vi "main double species.vi"() -> ()   [LabVIEW 2013]
uses:
  <vilib>/Utility/file.llb/Read From Spreadsheet File (DBL).vi
panel:
  out "Process Index":i8
  out "XY图 4":cluster{i32[], dbl[]}[](graph)
  out "XY图 3":cluster{i32[], dbl[]}[](graph)
  out "OD image 2":dbl[][](graph)
  out "Latest image data 2":dbl[][](array[numeric])
  out "Process Index 2":i8
  out "Two Cameras？":bool
  in  "Fitting Results Save Path 2":string[](array[string])
  in  "Fitting Type 2":u8(ring)
  in  "Force Guess? 2":bool
  in  "Initial guess values 2":dbl[](array[numeric])
  out "From OD fit?":bool
  in  "Current file num":i32
  in  "Fitting Results Save Path":string[](array[string])
  in  "Initial guess values":dbl[](array[numeric])
  out "Latest image data":dbl[][](array[numeric])
  in  "Fitting Type":u8(ring)
  in  "Force Guess?":bool
  out "Fit Done 2":bool
  out "ROI Width 2":u16
  out "ROI Height 2":u16
  out "External Trigger 2":bool
  in  "Fitting Config 2":bool
  in  "Camera Config 2":bool
  in  "Camera2":refnum<k7>(container)
  out "ROI Height":u16
  out "ROI Width":u16
  out "OD image":dbl[][](graph)
  out "External Trigger":bool
  out "XY图":cluster{i32[], dbl[]}[](graph)
  in  "OD fit":bool
  in  "OD num":i32
  out "Fit Done":bool
  in  "Exit":bool
  out "XY图 2":cluster{i32[], dbl[]}[](graph)
  in  "Auto Split":bool
  in  "Fit":bool
  in  "Open File":bool
  in  "Auto Fit":bool
  in  "Stop":bool
  in  "Aquire":bool
  in  "Fitting Config 1":bool
  in  "Camera Config 1":bool
  in  "Initialize":bool
  in  "Camera1":refnum<k7>(container)
  # "Camera Config"
  # "Fitting Config"
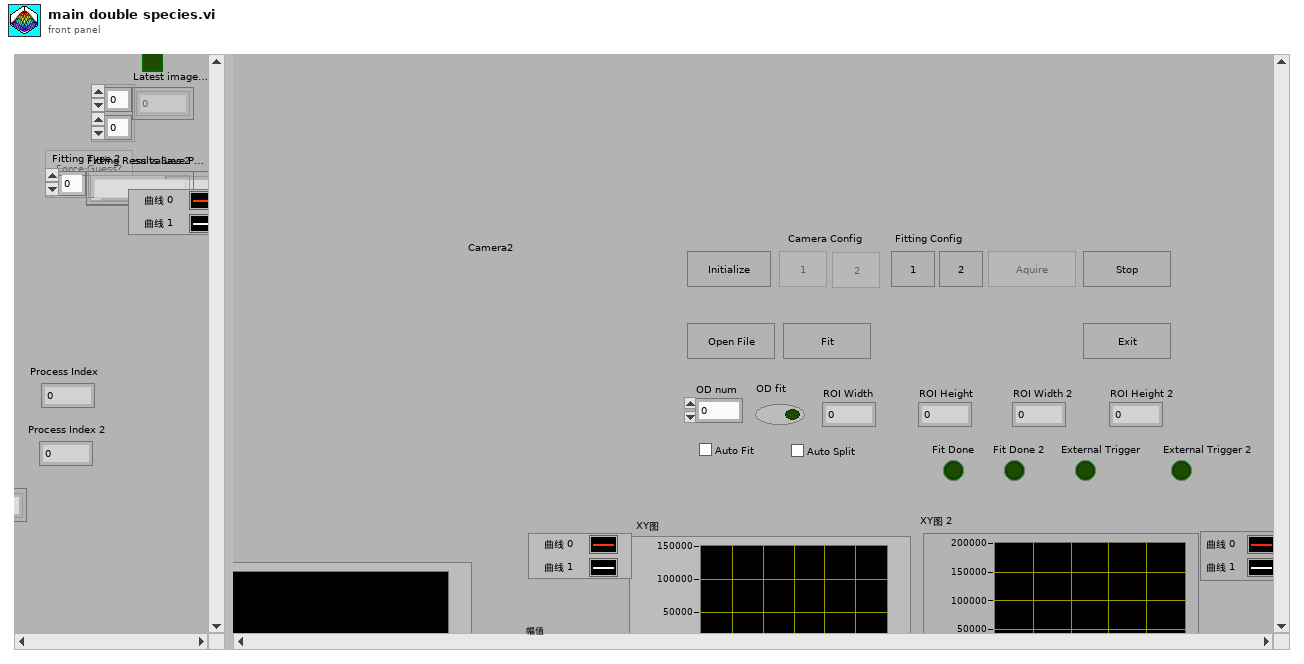
[diagram p1: front panel]
types:
  T1 = enum8{"Enabled", "Disabled", "Disabled and Grayed Out"}
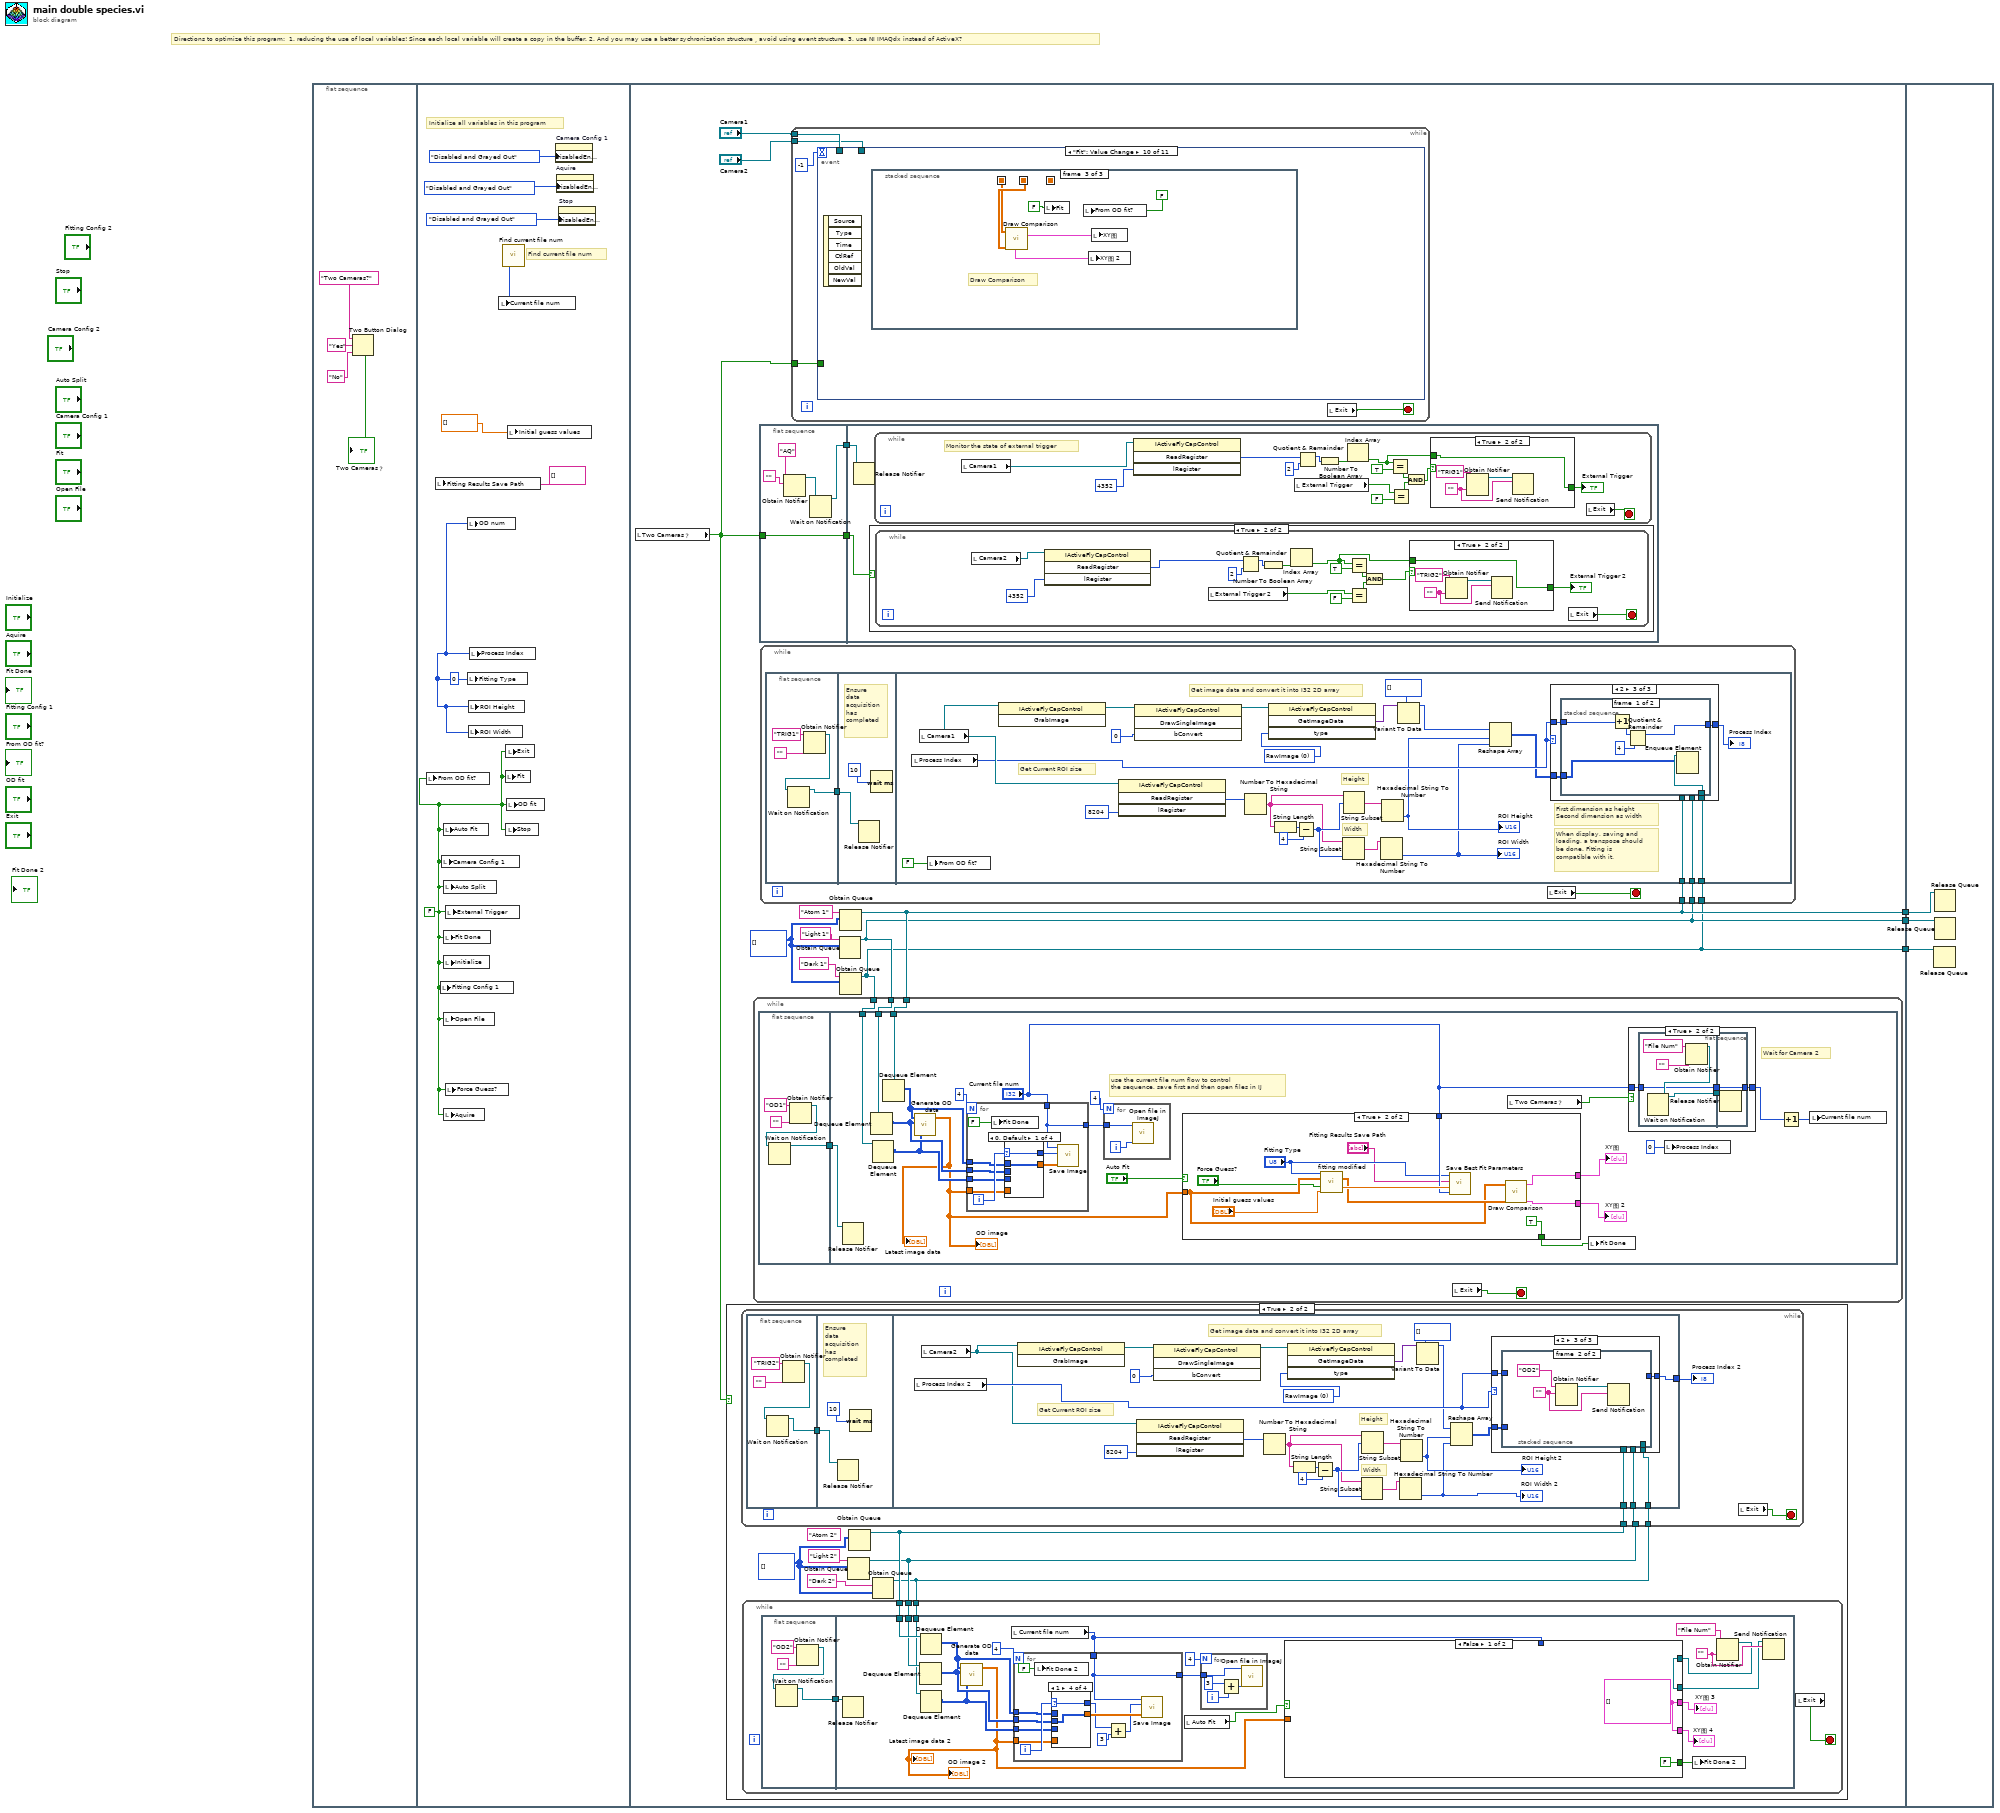
[diagram p0: block diagram]
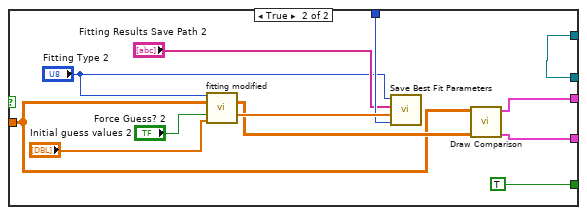
[diagram p3: hidden frame]
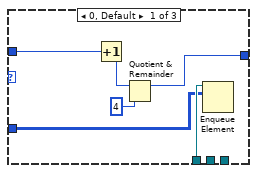
[diagram p7: hidden frame]
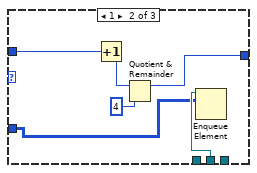
[diagram p8: hidden frame]
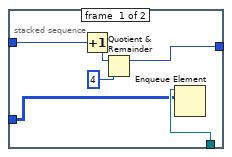
[diagram p9: hidden frame]
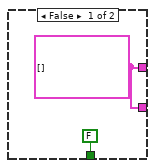
[diagram p11: hidden frame]
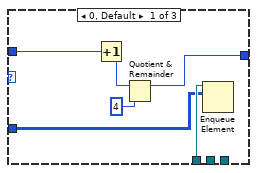
[diagram p18: hidden frame]
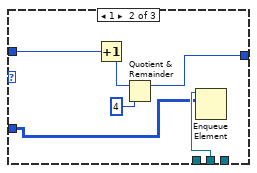
[diagram p19: hidden frame]
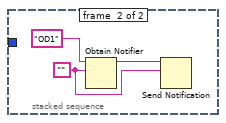
[diagram p20: hidden frame]
diagram:
  # "Directions to optimize this program:  1. reducing the use of local variables! Since each local variable will create a copy in the buffer. 2. And you may use a better sychronization structure，avoid using event structure. 3. use NI IMAQdx instead of ActiveX?"
  n1 = flat-sequence {
    tunnel: [w22] -> w3
    tunnel: [w21] -> w2
    tunnel: [w20] -> w1
    tunnel: w3 -> [w446]
    tunnel: w2 -> [w445]
    tunnel: w1 -> [w444]
    frame #0 {
      n2 = Two Button Dialog(message="Two Cameras?" ("消息"), 1:"No" ("F按钮名称（“取消”）"), 2:"Yes" ("T按钮名称（“确定”）")) -> (T button?=→"Two Cameras？":bool)
    }
    frame #1 {
      w11 = 0 ("OD num")
      w9 = FALSE ("Aquire")
      # "Find current file num"
      # "Initialize all variables in this program"
      n3 = local write "From OD fit?"(w9) -> ()
      n4 = local write "Fitting Results Save Path"(string[] [] ("Fitting Results Save Path")) -> ()
      n5 = local write "Fitting Config 1"(w9) -> ()
      n6 = local write "Camera Config 1"(w9) -> ()
      n7 = local write "Auto Fit"(w9) -> ()
      n8 = local write "Auto Split"(w9) -> ()
      n9 = local write "Fit Done"(w9) -> ()
      n10 = local write "Initialize"(w9) -> ()
      n11 = local write "Open File"(w9) -> ()
      n12 = local write "Aquire"(w9) -> ()
      n13 = local write "Force Guess?"(w9) -> ()
      n14 = local write "External Trigger"(w9) -> ()
      n15 = local write "OD num"(w11) -> ()
      n16 = local write "Fitting Type"(w11) -> ()
      n17 = local write "ROI Height"(w11) -> ()
      n18 = local write "ROI Width"(w11) -> ()
      n19 = local write "Process Index"(w11) -> ()
      n20 = call "Find current file num.vi"() -> ("Current File Num"=w8:u16)  [unwired: 2 in]
      n21 = local write "Current file num"(w8) -> ()
      n22 = local write "Fit"(w9) -> ()
      n23 = local write "Exit"(w9) -> ()
      n24 = local write "Stop"(w9) -> ()
      n25 = local write "OD fit"(w9) -> ()
      n26 = local write "Initial guess values"(dbl[] [] ("Best fit parameters")) -> ()
      n27 = property on="Camera Config 1" class="Bool (strict)"("DisabledEnum"=T1."Disabled and Grayed Out" ("禁用")) -> ()  [unwired: 2 in, 2 out]
      n28 = property on="Aquire" class="Bool (strict)"("DisabledEnum"=T1."Disabled and Grayed Out" ("禁用")) -> ()  [unwired: 2 in, 2 out]
      n29 = property on="Stop" class="Bool (strict)"("DisabledEnum"=T1."Disabled and Grayed Out" ("禁用")) -> ()  [unwired: 2 in, 2 out]
    }
    frame #2 {
      w23 = u16[][] [] ("输出数组")
      n30 = local read "Two Cameras？"() -> (w16:bool)
      n31 = case shown="True" w16 {
        frame False {
        }
        frame True {
          w31 = u16[][] [] ("输出数组")
          (unwired) "Atom 2" ("名称（未命名）")
          n32 = Obtain Queue(name (unnamed)="Light 2" ("名称（未命名）"), element data type=w31) -> (queue out=w29:refnum<queue>)  [unwired: 3 in, 2 out]
          n33 = Obtain Queue(element data type=w31) -> (queue out=w30:refnum<queue>)  [unwired: 4 in, 2 out]
          n34 = Obtain Queue(name (unnamed)="Dark 2" ("名称（未命名）"), element data type=w31) -> (queue out=w28:refnum<queue>)  [unwired: 3 in, 2 out]
          n35 = while {
            tunnel: w30 -> [w103]
            tunnel: w29 -> [w102]
            tunnel: w28 -> [w101]
            stop <- w104 stop-if-true
            n36 = flat-sequence {
              tunnel: [w107] -> w106
              tunnel: w106 -> [w111]
              tunnel: [w122] -> w105
              tunnel: w103 -> [w115]
              tunnel: w102 -> [w114]
              tunnel: w101 -> [w113]
              frame #0 {
                n37 = Obtain Notifier(name (unnamed)="TRIG2" ("名称（未命名）"), notification data type="") -> (notifier out=w108:refnum<notifier>)  [unwired: 2 in, 2 out]
                n38 = Wait on Notification(notifier=w108) -> (notifier out=w107:refnum<notifier>)  [unwired: 3 in, 3 out]
              }
              frame #1 {
                # "Ensure\ndata\nacquisition\nhas \ncompleted"
                n39 = Release Notifier(notifier=w111) -> ()  [unwired: 2 in, 3 out]
                n40 = Wait (ms)(milliseconds to wait=u32 10 ("等待时间（毫秒）")) -> ()  [unwired: 1 out]
              }
              frame #2 {
                w136 = 0 items=["RawImage", "ColorProcessedImage"] ("type")
                # "Get image data and convert it into I32 2D array"
                # "Width"
                # "Height"
                # "Get Current ROI size"
                n41 = local read "Process Index 2"() -> (w121:i8)
                n42 = local read "Camera2"() -> (w116:refnum<k7>)
                n43 = invoke class="IActiveFlyCapControl" method="GrabImage"(reference=w116) -> (reference out=w125:refnum<k7>)  [unwired: 2 in, 2 out]
                n44 = invoke class="IActiveFlyCapControl" method="ReadRegister"(reference=w116, "lRegister"=u32 8204) -> ("ReadRegister"=w133:u32)  [unwired: 2 in, 3 out]
                n45 = invoke class="IActiveFlyCapControl" method="DrawSingleImage"(reference=w125, "bConvert"=0) -> (reference out=w126:refnum<k7>)  [unwired: 2 in, 3 out]
                n46 = Number To Hexadecimal String(2:w133) -> (0:w129:string)  [unwired: 1 in]
                n47 = invoke class="IActiveFlyCapControl" method="GetImageData"(reference=w126, "type"=w136) -> ("GetImageData"=w134:variant)  [unwired: 2 in, 3 out]
                n48 = String Length(string=w129) -> (length=w132:i32)
                n49 = Subtract(x=w132, y=4) -> (x-y=w130:i32)
                n50 = String Subset(string=w129, length (rest)=w130) -> (substring=w127:string)  [unwired: 1 in]
                n51 = String Subset(string=w129, offset (0)=w130) -> (substring=w128:string)  [unwired: 1 in]
                n52 = Hexadecimal String To Number(string=w127) -> (number=w119:u32)  [unwired: 2 in, 1 out]
                "ROI Width 2" <- w119
                n53 = Hexadecimal String To Number(string=w128) -> (number=w120:u32)  [unwired: 2 in, 1 out]
                "ROI Height 2" <- w120
                n54 = Variant To Data(type=u16[] [], Variant=w134) -> (data=w118:u16[])  [unwired: 1 in, 1 out]
                n55 = Reshape Array(w118, w120, w119) -> (w117:u16[][])
                n56 = case shown="2" w121 {
                  tunnel: w121 -> [w140 w146 w152]
                  tunnel: w117 -> [w138 w144 w151]
                  tunnel: w115 -> [w139 _ _]
                  tunnel: w114 -> [_ w145 _]
                  tunnel: w113 -> [_ _ w150]
                  tunnel: [w137 w143 w149] -> w122
                  frame 0, Default {
                    n57 = Increment(x=w140) -> (x+1=w141:i8)
                    n58 = Quotient & Remainder(x=w141, y=4) -> (x-y*floor(x/y)=w137:i32)  [unwired: 1 out]
                    n59 = Enqueue Element(queue=w139, element=w138) -> ()  [unwired: 2 in, 3 out]
                  }
                  frame 1 {
                    n60 = Increment(x=w146) -> (x+1=w147:i8)
                    n61 = Quotient & Remainder(x=w147, y=4) -> (x-y*floor(x/y)=w143:i32)  [unwired: 1 out]
                    n62 = Enqueue Element(queue=w145, element=w144) -> ()  [unwired: 2 in, 3 out]
                  }
                  frame 2 {
                    n63 = stacked-sequence {
                      tunnel: w152 -> [w156 _]
                      tunnel: w151 -> [w154 _]
                      tunnel: w150 -> [w155 _]
                      tunnel: [w153 _] -> w149
                      frame #0 {
                        n64 = Increment(x=w156) -> (x+1=w157:i8)
                        n65 = Quotient & Remainder(x=w157, y=4) -> (x-y*floor(x/y)=w153:i32)  [unwired: 1 out]
                        n66 = Enqueue Element(queue=w155, element=w154) -> ()  [unwired: 2 in, 3 out]
                      }
                      frame #1 {
                        w159 = ""
                        n67 = Obtain Notifier(name (unnamed)="OD2" ("名称（未命名）"), notification data type=w159) -> (notifier out=w161:refnum<notifier>)  [unwired: 2 in, 2 out]
                        n68 = Send Notification(notification=w159, notifier=w161) -> ()  [unwired: 1 in, 2 out]
                      }
                    }
                  }
                }
              }
            }
            n69 = local read "Exit"() -> (w104:bool)
            "Process Index 2" <- w105
          }
          n70 = while {
            tunnel: w30 -> [w37]
            tunnel: w29 -> [w36]
            tunnel: w28 -> [w35]
            stop <- w34 stop-if-true
            n71 = flat-sequence {
              tunnel: [w39] -> w38
              tunnel: w38 -> [w62]
              tunnel: w37 -> [w57]
              tunnel: w36 -> [w56]
              tunnel: w35 -> [w55]
              frame #0 {
                n72 = Obtain Notifier(name (unnamed)="OD2" ("名称（未命名）"), notification data type="") -> (notifier out=w40:refnum<notifier>)  [unwired: 2 in, 2 out]
                n73 = Wait on Notification(notifier=w40) -> (notifier out=w39:refnum<notifier>)  [unwired: 3 in, 3 out]
              }
              frame #1 {
                w46 = ""
                n74 = Release Notifier(notifier=w62) -> ()  [unwired: 2 in, 3 out]
                n75 = Dequeue Element(queue=w56) -> (element=w59:u16[][])  [unwired: 2 in, 3 out]
                n76 = Dequeue Element(queue=w57) -> (element=w60:u16[][])  [unwired: 2 in, 3 out]
                n77 = Dequeue Element(queue=w55) -> (element=w58:u16[][])  [unwired: 2 in, 3 out]
                n78 = call "Generate OD data.vi"("dark"=w58, "light"=w59, "atom"=w60) -> ("OD image"=w52:dbl[][])  [unwired: 3 in]
                "Latest image data 2" <- w52
                "OD image 2" <- w52
                n79 = local read "Current file num"() -> (w50:i32)
                n80 = for {
                  N: 4 -> [_]
                  tunnel: w60 -> [w91]
                  tunnel: w59 -> [w90]
                  tunnel: w58 -> [w89]
                  tunnel: w52 -> [w88]
                  tunnel: w50 -> [w86]
                  tunnel: [w86] -> w53
                  i -> [w92]
                  n81 = local write "Fit Done 2"(FALSE ("Fit Done 2")) -> ()
                  n82 = case shown="1" w92 {
                    selector: w92 -> [w94 w96 w98 w100]
                    tunnel: w91 -> [w93 _ _ _]
                    tunnel: w90 -> [_ _ _ w99]
                    tunnel: w89 -> [_ w95 _ _]
                    tunnel: w88 -> [_ _ w97 _]
                    tunnel: [w94 w96 w98 w100] -> w85
                    tunnel: [w93 w95 w97 w99] -> w87
                    frame 0, Default {
                    }
                    frame 2 {
                    }
                    frame 3 {
                    }
                    frame 1 {
                    }
                  }
                  n83 = Add(x=w85, y=3 ("x")) -> (x+y=w84:i32)
                  n84 = call "Save Image.vi"("Data"=w87, "Process Index"=w84, "Current File Num"=w86) -> ()  [unwired: 9 in]
                }
                n85 = local read "Auto Fit"() -> (w51:bool)
                n86 = for {
                  N: 4 -> [_]
                  tunnel: w53 -> [w81]
                  i -> [w79]
                  n87 = Add(x=i8 3, y=w79) -> (x+y=w78:i32)
                  n88 = call "Open file in ImageJ.vi"("Process Index"=w78, "Current File Num"=w81) -> ()  [unwired: 10 in]
                }
                n89 = Obtain Notifier(name (unnamed)="File Num" ("名称（未命名）"), notification data type=w46) -> (notifier out=w45:refnum<notifier>)  [unwired: 2 in, 2 out]
                n90 = case shown="False" w51 {
                  tunnel: w52 -> [_ w74]
                  tunnel: w50 -> [_ w76]
                  tunnel: [w65 w73] -> w49
                  tunnel: [w65 w72] -> w48
                  tunnel: w45 -> [w64 w67]
                  tunnel: [w64 w67] -> w44
                  tunnel: [FALSE ("Fit Done 2") TRUE ("Fit Done 2")] -> w43
                  frame False {
                    w65 = cluster{i32[], dbl[]}[] [] ("Horizontal Comparison")
                  }
                  frame True {
                    n91 = call "fitting modified.vi"("fitting type"="Fitting Type 2", "2D data"=w74, "force guess?"="Force Guess? 2", "intial guess value"="Initial guess values 2") -> ("best fit"=w75:dbl[][], "best fit parameters"=w77:dbl[])  [unwired: 9 in, 1 out]
                    n92 = call "Save Best Fit Parameters.vi"("Current File Num"=w76, "Best Fit Parameters"=w77, "Fitting Results Save Path"="Fitting Results Save Path 2", "Fitting Type"="Fitting Type 2") -> ()  [unwired: 8 in]
                    n93 = call "Draw Comparison.vi"("Best Fit"=w75, "Raw Data"=w74) -> ("Vertical Comparison"=w72:cluster{i32[], dbl[]}[], "Horizontal Comparison"=w73:cluster{i32[], dbl[]}[])  [unwired: 7 in]
                  }
                }
                "XY图 3" <- w49
                "XY图 4" <- w48
                n94 = local write "Fit Done 2"(w43) -> ()
                n95 = Send Notification(notification=w46, notifier=w44) -> ()  [unwired: 1 in, 2 out]
              }
            }
            n96 = local read "Exit"() -> (w34:bool)
          }
        }
      }
      n97 = flat-sequence {
        tunnel: [w236] -> w27
        tunnel: w16 -> [w235]
        tunnel: [w235] -> w17
        tunnel: w27 -> [w241]
        tunnel: w17 -> [w240]
        frame #0 {
          n98 = Obtain Notifier(name (unnamed)="AQ" ("名称（未命名）"), notification data type="") -> (notifier out=w238:refnum<notifier>)  [unwired: 2 in, 2 out]
          n99 = Wait on Notification(notifier=w238) -> (notifier out=w236:refnum<notifier>)  [unwired: 3 in, 3 out]
        }
        frame #1 {
          n100 = Release Notifier(notifier=w241) -> ()  [unwired: 2 in, 3 out]
          n101 = case shown="True" w240 {
            frame False {
            }
            frame True {
              n102 = while {
                stop <- w256 stop-if-true
                n103 = local read "Camera2"() -> (w242:refnum<k7>)
                n104 = invoke class="IActiveFlyCapControl" method="ReadRegister"(reference=w242, "lRegister"=u32 4352) -> ("ReadRegister"=w243:u32)  [unwired: 2 in, 3 out]
                n105 = local read "External Trigger 2"() -> (w245:bool)
                n106 = Quotient & Remainder(x=w243, y=u32 2) -> (x-y*floor(x/y)=w249:u32)  [unwired: 1 out]
                n107 = Number To Boolean Array(number=w249) -> (Boolean array=w248:bool[])
                n108 = Index Array(array=w248) -> (element=w247:bool)  [unwired: 1 in]
                n109 = Equal?(x=w247, y=TRUE) -> (x = y?=w252:bool)
                n110 = Equal?(x=w245, y=FALSE) -> (x = y?=w253:bool)
                n111 = And(x=w252, y=w253) -> (x .and. y?=w251:bool)
                n112 = case shown="True" w251 {
                  tunnel: w247 -> [w257 w258]
                  tunnel: [w257 w258] -> w246
                  frame False {
                  }
                  frame True {
                    w259 = ""
                    n113 = Obtain Notifier(name (unnamed)="TRIG2" ("名称（未命名）"), notification data type=w259) -> (notifier out=w260:refnum<notifier>)  [unwired: 2 in, 2 out]
                    n114 = Send Notification(notification=w259, notifier=w260) -> ()  [unwired: 1 in, 2 out]
                  }
                }
                "External Trigger 2" <- w246
                n115 = local read "Exit"() -> (w256:bool)
              }
            }
          }
          n116 = while {
            stop <- w276 stop-if-true
            # "Monitor the state of external trigger"
            n117 = local read "Camera1"() -> (w275:refnum<k7>)
            n118 = invoke class="IActiveFlyCapControl" method="ReadRegister"(reference=w275, "lRegister"=u32 4352) -> ("ReadRegister"=w273:u32)  [unwired: 2 in, 3 out]
            n119 = local read "External Trigger"() -> (w268:bool)
            n120 = Quotient & Remainder(x=w273, y=u32 2) -> (x-y*floor(x/y)=w271:u32)  [unwired: 1 out]
            n121 = Number To Boolean Array(number=w271) -> (Boolean array=w270:bool[])
            n122 = Index Array(array=w270) -> (element=w263:bool)  [unwired: 1 in]
            n123 = Equal?(x=w263, y=TRUE) -> (x = y?=w265:bool)
            n124 = Equal?(x=w268, y=FALSE) -> (x = y?=w266:bool)
            n125 = And(x=w265, y=w266) -> (x .and. y?=w264:bool)
            n126 = case shown="True" w264 {
              tunnel: w263 -> [w277 w278]
              tunnel: [w277 w278] -> w262
              frame False {
              }
              frame True {
                w279 = ""
                n127 = Obtain Notifier(name (unnamed)="TRIG1" ("名称（未命名）"), notification data type=w279) -> (notifier out=w280:refnum<notifier>)  [unwired: 2 in, 2 out]
                n128 = Send Notification(notification=w279, notifier=w280) -> ()  [unwired: 1 in, 2 out]
              }
            }
            "External Trigger" <- w262
            n129 = local read "Exit"() -> (w276:bool)
          }
        }
      }
      n130 = while {
        tunnel: "Camera1" -> [w346]
        tunnel: "Camera2" -> [w345]
        tunnel: w16 -> [w343]
        stop <- w347 stop-if-true
        n131 = event shown="[9] \"Fit\": Value Change" {
          selector: _ -> [_ _ _ _ _ _ _ _ _ _ _]
          dyn-events: _ -> [_ _ _ _ _ _ _ _ _ _ _]
          timeout: -1 -> [_ _ _ _ _ _ _ _ _ _ _]
          tunnel: w346 -> [_ w355 w374 _ _ _ _ w396 w411 _ _]
          tunnel: w345 -> [_ w354 _ w377 _ _ _ w397 w413 _ _]
          tunnel: w343 -> [_ w352 _ w376 _ w386 _ w394 w409 _ _]
          event "OD fit": Value Change {
            n132 = event-data() -> ()  [unwired: 1 in, 6 out]
            n133 = local write "OD fit"(FALSE ("OD fit")) -> ()
            n134 = call "Read OD data.vi"("OD num"="OD num") -> ("OD data"=w349:dbl[][])  [unwired: 4 in]
            n135 = local write "Latest image data"(w349) -> ()
            n136 = local write "OD image"(w349) -> ()
            n137 = local write "From OD fit?"(TRUE ("From OD fit?")) -> ()
          }
          event "Initialize": Value Change {
            w361 = 2 items=["FreeRunning", "LockNext", "LockLatest"] ("mode")
            # "Setup Camera Index"
            # "Set grab mode"
            # "Make Sure the camera is not running"
            n138 = event-data() -> ()  [unwired: 1 in, 6 out]
            n139 = case shown="True" w352 {
              tunnel: w354 -> [_ w369]
              frame False {
              }
              frame True {
                w366 = 2 items=["FreeRunning", "LockNext", "LockLatest"] ("mode")
                n140 = property class="IActiveFlyCapControl"(reference=w369, "Camera"=u32 1) -> (reference out=w368:refnum<k7>)  [unwired: 1 in, 1 out]
                n141 = invoke class="IActiveFlyCapControl" method="ShowCamSlnModal"(reference=w368) -> (reference out=w367:refnum<k7>)  [unwired: 2 in, 2 out]
                n142 = property class="IActiveFlyCapControl"(reference=w367, "Start"=0 ("Camera")) -> (reference out=w371:refnum<k7>)  [unwired: 1 in, 1 out]
                n143 = invoke class="IActiveFlyCapControl" method="SetGrabMode"(reference=w371, "mode"=w366) -> (reference out=w365:refnum<k7>)  [unwired: 2 in, 3 out]
                n144 = local write "Camera2"(w365) -> ()
              }
            }
            n145 = property class="IActiveFlyCapControl"(reference=w355, "Camera"=u32 0) -> (reference out=w360:refnum<k7>)  [unwired: 1 in, 1 out]
            n146 = invoke class="IActiveFlyCapControl" method="ShowCamSlnModal"(reference=w360) -> (reference out=w358:refnum<k7>)  [unwired: 2 in, 2 out]
            n147 = property class="IActiveFlyCapControl"(reference=w358, "Start"=0 ("Camera")) -> (reference out=w357:refnum<k7>)  [unwired: 1 in, 1 out]
            n148 = invoke class="IActiveFlyCapControl" method="SetGrabMode"(reference=w357, "mode"=w361) -> (reference out=w353:refnum<k7>)  [unwired: 2 in, 3 out]
            n149 = local write "Camera1"(w353) -> ()
            n150 = property on="Camera Config 1" class="Bool (strict)"("DisabledEnum"=T1."Enabled" ("禁用")) -> ()  [unwired: 2 in, 2 out]
            n151 = local write "Initialize"(FALSE ("Initialize")) -> ()
            n152 = property on="Aquire" class="Bool (strict)"("DisabledEnum"=T1."Enabled" ("禁用")) -> ()  [unwired: 2 in, 2 out]
          }
          event "Camera Config 1": Value Change {
            n153 = event-data() -> ()  [unwired: 1 in, 6 out]
            n154 = invoke class="IActiveFlyCapControl" method="ToggleCamCtlDlg"(reference=w374) -> (reference out=w373:refnum<k7>)  [unwired: 2 in, 2 out]
            n155 = local write "Camera Config 1"(FALSE ("Camera Config")) -> ()
            n156 = local write "Camera1"(w373) -> ()
          }
          event "Camera Config 2": Value Change {
            n157 = event-data() -> ()  [unwired: 1 in, 6 out]
            n158 = case shown="True" w376 {
              tunnel: w377 -> [_ w379]
              frame False {
              }
              frame True {
                n159 = invoke class="IActiveFlyCapControl" method="ToggleCamCtlDlg"(reference=w379) -> (reference out=w378:refnum<k7>)  [unwired: 2 in, 2 out]
                n160 = local write "Camera Config 2"(FALSE ("Camera Config 2")) -> ()
                n161 = local write "Camera2"(w378) -> ()
              }
            }
          }
          event "Fitting Config 1": Value Change {
            # "pump out fitting config. and transfer parameters"
            n162 = event-data() -> ()  [unwired: 1 in, 6 out]
            n163 = call "Fitting Configuration.vi"() -> ("intial guess"=w381:dbl[], "Force Guess？"=w382:bool, "Fitting Type"=w384:u16, "Fitting Results Save Path"=w383:string[])  [unwired: 5 in]
            n164 = local write "Fitting Results Save Path"(w383) -> ()
            n165 = local write "Fitting Type"(w384) -> ()
            n166 = local write "Fitting Config 1"(FALSE ("Fitting Config")) -> ()
            n167 = local write "Initial guess values"(w381) -> ()
            n168 = local write "Force Guess?"(w382) -> ()
          }
          event "Fitting Config 2": Value Change {
            n169 = event-data() -> ()  [unwired: 1 in, 6 out]
            n170 = case shown="True" w386 {
              frame False {
              }
              frame True {
                n171 = call "Fitting Configuration 2.vi"() -> ("intial guess"=w388:dbl[], "Force Guess？"=w389:bool, "Fitting Type"=w390:u16, "Fitting Results Save Path"=w391:string[])  [unwired: 5 in]
                n172 = local write "Initial guess values 2"(w388) -> ()
                n173 = local write "Force Guess? 2"(w389) -> ()
                n174 = local write "Fitting Results Save Path 2"(w391) -> ()
                n175 = local write "Fitting Type 2"(w390) -> ()
              }
            }
            n176 = local write "Fitting Config 2"(FALSE ("Fitting Config 2")) -> ()
          }
          event "Open File": Value Change {
            n177 = event-data() -> ()  [unwired: 1 in, 6 out]
            n178 = call-poly <vilib>:"Read From Spreadsheet File.vi"() -> ("all rows"=w392:dbl[][])  [unwired: 7 in, 4 out]
            n179 = local write "Open File"(FALSE ("Open File")) -> ()
            n180 = local write "OD image"(w392) -> ()
            n181 = local write "Latest image data"(w392) -> ()
          }
          event "Aquire": Value Change {
            w398 = 1 ("Start")
            w399 = ""
            # "Start the camera"
            n182 = event-data() -> ()  [unwired: 1 in, 6 out]
            n183 = case shown="True" w394 {
              tunnel: w398 -> [_ w408]
              tunnel: w397 -> [_ w407]
              frame False {
              }
              frame True {
                n184 = property class="IActiveFlyCapControl"(reference=w407, "Start"=w408) -> (reference out=w406:refnum<k7>)  [unwired: 1 in, 1 out]
                n185 = local write "Camera2"(w406) -> ()
              }
            }
            n186 = property class="IActiveFlyCapControl"(reference=w396, "Start"=w398) -> (reference out=w395:refnum<k7>)  [unwired: 1 in, 1 out]
            n187 = Obtain Notifier(name (unnamed)="AQ" ("名称（未命名）"), notification data type=w399) -> (notifier out=w400:refnum<notifier>)  [unwired: 2 in, 2 out]
            n188 = Send Notification(notification=w399, notifier=w400) -> ()  [unwired: 1 in, 2 out]
            n189 = local write "Camera1"(w395) -> ()
            n190 = property on="Aquire" class="Bool (strict)"("DisabledEnum"=T1."Disabled and Grayed Out" ("禁用")) -> ()  [unwired: 2 in, 2 out]
            n191 = property on="Stop" class="Bool (strict)"("DisabledEnum"=T1."Enabled" ("禁用")) -> ()  [unwired: 2 in, 2 out]
            n192 = property on="Camera Config 1" class="Bool (strict)"("DisabledEnum"=T1."Disabled and Grayed Out" ("禁用")) -> ()  [unwired: 2 in, 2 out]
            n193 = local write "Aquire"(FALSE ("Initialize")) -> ()
          }
          event "Stop": Value Change {
            w412 = 0 ("Start")
            # "stop the camera"
            n194 = event-data() -> ()  [unwired: 1 in, 6 out]
            n195 = case shown="True" w409 {
              tunnel: w413 -> [_ w419]
              tunnel: w412 -> [_ w418]
              frame False {
              }
              frame True {
                n196 = property class="IActiveFlyCapControl"(reference=w419, "Start"=w418) -> (reference out=w417:refnum<k7>)  [unwired: 1 in, 1 out]
                n197 = local write "Camera2"(w417) -> ()
              }
            }
            n198 = property class="IActiveFlyCapControl"(reference=w411, "Start"=w412) -> (reference out=w410:refnum<k7>)  [unwired: 1 in, 1 out]
            n199 = local write "Camera1"(w410) -> ()
            n200 = local write "Stop"(FALSE ("Initialize")) -> ()
            n201 = property on="Stop" class="Bool (strict)"("DisabledEnum"=T1."Disabled and Grayed Out" ("禁用")) -> ()  [unwired: 2 in, 2 out]
            n202 = property on="Aquire" class="Bool (strict)"("DisabledEnum"=T1."Enabled" ("禁用")) -> ()  [unwired: 2 in, 2 out]
          }
          event "Fit": Value Change {
            n203 = event-data() -> ()  [unwired: 1 in, 6 out]
            n204 = stacked-sequence {
              seq-local: [w421 _ _] -> [_ _ w440]
              seq-local: [w422 _ _] -> [_ _ w438]
              seq-local: [w420 _ _] -> [_ w431 _]
              frame #0 {
                n205 = flat-sequence {
                  tunnel: [w425] -> w422
                  tunnel: [w424] -> w421
                  tunnel: [w423] -> w420
                  frame #0 {
                    # "Fit the latest data"
                    n206 = local read "Latest image data"() -> (w425:dbl[][])
                    n207 = local read "Initial guess values"() -> (w427:dbl[])
                    n208 = local read "Force Guess?"() -> (w428:bool)
                    n209 = local read "Fitting Type"() -> (w426:u8)
                    n210 = call "fitting modified.vi"("fitting type"=w426, "2D data"=w425, "force guess?"=w428, "intial guess value"=w427) -> ("best fit"=w424:dbl[][], "best fit parameters"=w423:dbl[])  [unwired: 9 in, 1 out]
                  }
                  frame #1 {
                    n211 = local write "Fit"(FALSE ("Fit")) -> ()
                    n212 = local write "Fit Done"(TRUE ("Fit Done")) -> ()
                  }
                }
              }
              frame #1 {
                # "Save best fit parameters"
                n213 = local read "Fitting Results Save Path"() -> (w434:string[])
                n214 = local read "Fitting Type"() -> (w435:u8)
                n215 = local read "From OD fit?"() -> (w433:bool)
                n216 = case shown="True" w433 {
                  tunnel: [w436 w437] -> w432
                  frame False {
                    n217 = local read "Current file num"() -> (w436:i32)
                  }
                  frame True {
                    n218 = local read "OD num"() -> (w437:i32)
                  }
                }
                n219 = call "Save Best Fit Parameters.vi"("Current File Num"=w432, "Best Fit Parameters"=w431, "Fitting Results Save Path"=w434, "Fitting Type"=w435) -> ()  [unwired: 8 in]
              }
              frame #2 {
                # "Draw Comparison"
                n220 = call "Draw Comparison.vi"("Best Fit"=w440, "Raw Data"=w438) -> ("Vertical Comparison"=w442:cluster{i32[], dbl[]}[], "Horizontal Comparison"=w443:cluster{i32[], dbl[]}[])  [unwired: 7 in]
                n221 = local write "Fit"(FALSE ("Initialize")) -> ()
                n222 = local write "From OD fit?"(FALSE ("From OD fit?")) -> ()
                n223 = local write "XY图 2"(w442) -> ()
                n224 = local write "XY图"(w443) -> ()
              }
            }
          }
          event Timeout {
            n225 = event-data() -> ()  [unwired: 1 in, 3 out]
          }
        }
        n226 = local read "Exit"() -> (w347:bool)
      }
      n227 = Obtain Queue(name (unnamed)="Light 1" ("名称（未命名）"), element data type=w23) -> (queue out=w21:refnum<queue>)  [unwired: 3 in, 2 out]
      n228 = Obtain Queue(name (unnamed)="Atom 1" ("名称（未命名）"), element data type=w23) -> (queue out=w22:refnum<queue>)  [unwired: 3 in, 2 out]
      n229 = Obtain Queue(name (unnamed)="Dark 1" ("名称（未命名）"), element data type=w23) -> (queue out=w20:refnum<queue>)  [unwired: 3 in, 2 out]
      n230 = while {
        tunnel: w22 -> [w164]
        tunnel: w21 -> [w163]
        tunnel: w20 -> [w162]
        stop <- w166 stop-if-true
        n231 = flat-sequence {
          tunnel: [w167] -> w165
          tunnel: w165 -> [w190]
          tunnel: w164 -> [w188]
          tunnel: w163 -> [w186]
          tunnel: w162 -> [w184]
          frame #0 {
            n232 = Obtain Notifier(name (unnamed)="OD1" ("名称（未命名）"), notification data type="") -> (notifier out=w168:refnum<notifier>)  [unwired: 2 in, 2 out]
            n233 = Wait on Notification(notifier=w168) -> (notifier out=w167:refnum<notifier>)  [unwired: 3 in, 3 out]
          }
          frame #1 {
            # "Wait for Camera 2"
            # "use the current file num flow to control \nthe sequence, save first and then open files in IJ"
            n234 = Release Notifier(notifier=w190) -> ()  [unwired: 2 in, 3 out]
            n235 = Dequeue Element(queue=w186) -> (element=w185:u16[][])  [unwired: 2 in, 3 out]
            n236 = Dequeue Element(queue=w184) -> (element=w183:u16[][])  [unwired: 2 in, 3 out]
            n237 = Dequeue Element(queue=w188) -> (element=w187:u16[][])  [unwired: 2 in, 3 out]
            n238 = call "Generate OD data.vi"("dark"=w183, "light"=w185, "atom"=w187) -> ("OD image"=w179:dbl[][])  [unwired: 3 in]
            "OD image" <- w179
            "Latest image data" <- w179
            n239 = for {
              N: 4 -> [_]
              tunnel: w187 -> [w225]
              tunnel: w185 -> [w224]
              tunnel: w183 -> [w223]
              tunnel: w179 -> [w222]
              tunnel: "Current file num" -> [w219]
              tunnel: [w219] -> w177
              i -> [w226]
              n240 = local write "Fit Done"(FALSE ("Fit Done")) -> ()
              n241 = case shown="0, Default" w226 {
                selector: w226 -> [w228 w230 w232 w234]
                tunnel: w225 -> [w227 _ _ _]
                tunnel: w224 -> [_ _ _ w233]
                tunnel: w223 -> [_ w229 _ _]
                tunnel: w222 -> [_ _ w231 _]
                tunnel: [w228 w230 w232 w234] -> w221
                tunnel: [w227 w229 w231 w233] -> w220
                frame 0, Default {
                }
                frame 2 {
                }
                frame 3 {
                }
                frame 1 {
                }
              }
              n242 = call "Save Image.vi"("Data"=w220, "Process Index"=w221, "Current File Num"=w219) -> ()  [unwired: 9 in]
            }
            n243 = for {
              N: 4 -> [_]
              tunnel: w177 -> [w204]
              i -> [w203]
              n244 = call "Open file in ImageJ.vi"("Process Index"=w203, "Current File Num"=w204) -> ()  [unwired: 10 in]
            }
            n245 = case shown="True" "Auto Fit" {
              tunnel: w179 -> [_ w214]
              tunnel: "Current file num" -> [_ w216]
              tunnel: [w206 w213] -> w180
              tunnel: [w206 w212] -> w181
              tunnel: [FALSE ("Fit Done") TRUE ("Fit Done")] -> w171
              frame False {
                w206 = cluster{i32[], dbl[]}[] [] ("Horizontal Comparison")
              }
              frame True {
                n246 = call "fitting modified.vi"("fitting type"="Fitting Type", "2D data"=w214, "force guess?"="Force Guess?", "intial guess value"="Initial guess values") -> ("best fit"=w215:dbl[][], "best fit parameters"=w217:dbl[])  [unwired: 9 in, 1 out]
                n247 = call "Save Best Fit Parameters.vi"("Current File Num"=w216, "Best Fit Parameters"=w217, "Fitting Results Save Path"="Fitting Results Save Path", "Fitting Type"="Fitting Type") -> ()  [unwired: 8 in]
                n248 = call "Draw Comparison.vi"("Best Fit"=w215, "Raw Data"=w214) -> ("Vertical Comparison"=w212:cluster{i32[], dbl[]}[], "Horizontal Comparison"=w213:cluster{i32[], dbl[]}[])  [unwired: 7 in]
              }
            }
            "XY图" <- w180
            "XY图 2" <- w181
            n249 = local read "Two Cameras？"() -> (w174:bool)
            n250 = local write "Fit Done"(w171) -> ()
            n251 = case shown="True" w174 {
              tunnel: "Current file num" -> [w191 w195]
              tunnel: [w191 w194] -> w172
              frame False {
              }
              frame True {
                n252 = flat-sequence {
                  tunnel: w195 -> [w197]
                  tunnel: [w197] -> w193
                  tunnel: [w196] -> w192
                  tunnel: [w202] -> w194
                  tunnel: w193 -> [w202]
                  tunnel: w192 -> [w201]
                  frame #0 {
                    n253 = Obtain Notifier(name (unnamed)="File Num" ("名称（未命名）"), notification data type="") -> (notifier out=w198:refnum<notifier>)  [unwired: 2 in, 2 out]
                    n254 = Wait on Notification(notifier=w198) -> (notifier out=w196:refnum<notifier>)  [unwired: 3 in, 3 out]
                  }
                  frame #1 {
                    n255 = Release Notifier(notifier=w201) -> ()  [unwired: 2 in, 3 out]
                  }
                }
              }
            }
            n256 = local write "Process Index"(0 ("Process Index")) -> ()
            n257 = Increment(x=w172) -> (x+1=w173:i32)
            n258 = local write "Current file num"(w173) -> ()
          }
        }
        n259 = local read "Exit"() -> (w166:bool)
      }
      n260 = while {
        tunnel: w22 -> [w284]
        tunnel: w21 -> [w283]
        tunnel: w20 -> [w282]
        stop <- w286 stop-if-true
        n261 = flat-sequence {
          tunnel: [w287] -> w285
          tunnel: w285 -> [w292]
          tunnel: w284 -> [w296]
          tunnel: w283 -> [w295]
          tunnel: w282 -> [w294]
          frame #0 {
            n262 = Obtain Notifier(name (unnamed)="TRIG1" ("名称（未命名）"), notification data type="") -> (notifier out=w288:refnum<notifier>)  [unwired: 2 in, 2 out]
            n263 = Wait on Notification(notifier=w288) -> (notifier out=w287:refnum<notifier>)  [unwired: 3 in, 3 out]
          }
          frame #1 {
            # "Ensure\ndata\nacquisition\nhas \ncompleted"
            n264 = Release Notifier(notifier=w292) -> ()  [unwired: 2 in, 3 out]
            n265 = Wait (ms)(milliseconds to wait=u32 10 ("等待时间（毫秒）")) -> ()  [unwired: 1 out]
          }
          frame #2 {
            w317 = 0 items=["RawImage", "ColorProcessedImage"] ("type")
            # "Get image data and convert it into I32 2D array"
            # "When display, saving and \nloading, a transpose should\nbe done. Fitting is \ncompatible with it."
            # "First dimension as height\nSecond dimension as width"
            # "Width"
            # "Height"
            # "Get Current ROI size"
            n266 = local read "Process Index"() -> (w300:i8)
            n267 = local read "Camera1"() -> (w304:refnum<k7>)
            n268 = local write "From OD fit?"(FALSE ("From OD fit?")) -> ()
            n269 = invoke class="IActiveFlyCapControl" method="GrabImage"(reference=w304) -> (reference out=w302:refnum<k7>)  [unwired: 2 in, 2 out]
            n270 = invoke class="IActiveFlyCapControl" method="ReadRegister"(reference=w304, "lRegister"=u32 8204) -> ("ReadRegister"=w314:u32)  [unwired: 2 in, 3 out]
            n271 = invoke class="IActiveFlyCapControl" method="DrawSingleImage"(reference=w302, "bConvert"=0) -> (reference out=w303:refnum<k7>)  [unwired: 2 in, 3 out]
            n272 = Number To Hexadecimal String(2:w314) -> (0:w310:string)  [unwired: 1 in]
            n273 = invoke class="IActiveFlyCapControl" method="GetImageData"(reference=w303, "type"=w317) -> ("GetImageData"=w315:variant)  [unwired: 2 in, 3 out]
            n274 = String Length(string=w310) -> (length=w313:i32)
            n275 = Subtract(x=w313, y=4) -> (x-y=w311:i32)
            n276 = String Subset(string=w310, length (rest)=w311) -> (substring=w307:string)  [unwired: 1 in]
            n277 = String Subset(string=w310, offset (0)=w311) -> (substring=w308:string)  [unwired: 1 in]
            n278 = Hexadecimal String To Number(string=w307) -> (number=w297:u32)  [unwired: 2 in, 1 out]
            "ROI Width" <- w297
            n279 = Hexadecimal String To Number(string=w308) -> (number=w298:u32)  [unwired: 2 in, 1 out]
            "ROI Height" <- w298
            n280 = Variant To Data(type=u16[] [], Variant=w315) -> (data=w306:u16[])  [unwired: 1 in, 1 out]
            n281 = Reshape Array(w306, w298, w297) -> (w299:u16[][])
            n282 = case shown="2" w300 {
              tunnel: w300 -> [w321 w327 w333]
              tunnel: w299 -> [w319 w325 w332]
              tunnel: w296 -> [w320 _ _]
              tunnel: w295 -> [_ w326 _]
              tunnel: w294 -> [_ _ w331]
              tunnel: [w318 w324 w330] -> w293
              frame 0, Default {
                n283 = Increment(x=w321) -> (x+1=w322:i8)
                n284 = Quotient & Remainder(x=w322, y=4) -> (x-y*floor(x/y)=w318:i32)  [unwired: 1 out]
                n285 = Enqueue Element(queue=w320, element=w319) -> ()  [unwired: 2 in, 3 out]
              }
              frame 1 {
                n286 = Increment(x=w327) -> (x+1=w328:i8)
                n287 = Quotient & Remainder(x=w328, y=4) -> (x-y*floor(x/y)=w324:i32)  [unwired: 1 out]
                n288 = Enqueue Element(queue=w326, element=w325) -> ()  [unwired: 2 in, 3 out]
              }
              frame 2 {
                n289 = stacked-sequence {
                  tunnel: w333 -> [w337 _]
                  tunnel: w332 -> [w335 _]
                  tunnel: w331 -> [w336 _]
                  tunnel: [w334 _] -> w330
                  frame #0 {
                    n290 = Increment(x=w337) -> (x+1=w338:i8)
                    n291 = Quotient & Remainder(x=w338, y=4) -> (x-y*floor(x/y)=w334:i32)  [unwired: 1 out]
                    n292 = Enqueue Element(queue=w336, element=w335) -> ()  [unwired: 2 in, 3 out]
                  }
                  frame #1 {
                    w340 = ""
                    n293 = Obtain Notifier(name (unnamed)="OD1" ("名称（未命名）"), notification data type=w340) -> (notifier out=w342:refnum<notifier>)  [unwired: 2 in, 2 out]
                    n294 = Send Notification(notification=w340, notifier=w342) -> ()  [unwired: 1 in, 2 out]
                  }
                }
              }
            }
            "Process Index" <- w293
          }
        }
        n295 = local read "Exit"() -> (w286:bool)
      }
    }
    frame #3 {
      n296 = Release Queue(queue=w444) -> ()  [unwired: 2 in, 3 out]
      n297 = Release Queue(queue=w446) -> ()  [unwired: 2 in, 3 out]
      n298 = Release Queue(queue=w445) -> ()  [unwired: 2 in, 3 out]
    }
  }
